vi "Query Asset Utilization.vi"(8 "Error In":errorcluster, 9 "Utilization Filter":string, 10 "Asset Filter":string, 11 "Session In":refnum<class "NI Skyline Configuration HTTP.lvclass">) -> (0 "Error Out":errorcluster, 2 "Asset Utilization":T1(array[cluster]), 3 "Session Out":refnum<class "NI Skyline Configuration HTTP.lvclass">)   [LabVIEW 2020]
uses:
  <vilib>/Skyline/Configuration/Configuration HTTP_class/NI Skyline Configuration HTTP.lvclass
  <vilib>/Skyline/Configuration/Configuration HTTP_class/NI Skyline Configuration HTTP.lvclass/NI Skyline Configuration HTTP.ctl
  <vilib>/Skyline/Configuration/Configuration HTTP_class/Read Server URL.vi
  <vilib>/httpClient/POSTBuffer.vi
  <vilib>/httpClient/LabVIEWHTTPClient.lvlib
panel:
  out "Server URL":string
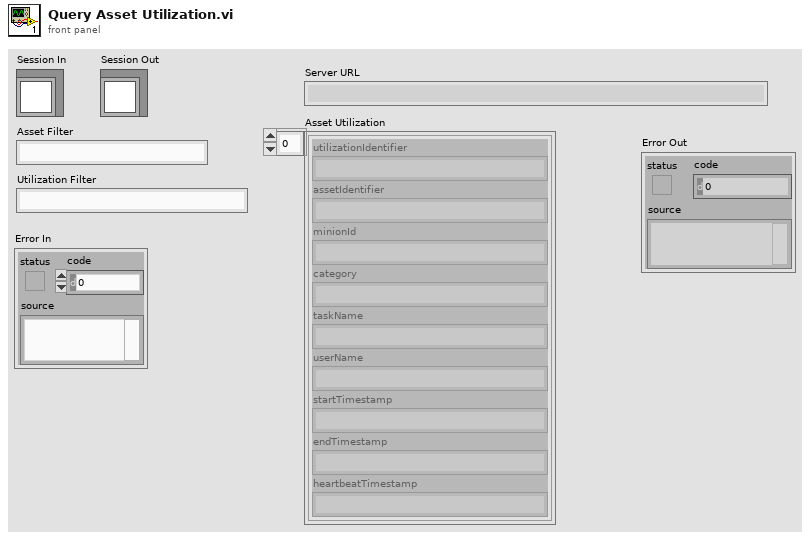
[diagram p1: front panel]
types:
  T1 = cluster{"utilizationIdentifier":string, "assetIdentifier":string, "minionId":string, "category":string, "taskName":string, "userName":string, "startTimestamp":string, "endTimestamp":string, "heartbeatTimestamp":string}[]
  T2 = cluster{"assetUtilizations":cluster{"utilizationIdentifier":string, "assetIdentifier":string, "minionId":string, "category":string, "taskName":string, "userName":string, "startTimestamp":string, "endTimestamp":string, "heartbeatTimestamp":string}[]}
  T3 = typedef "LabVIEWHTTPClient.lvlib/ClientHandle.ctl" = refnum<k1>
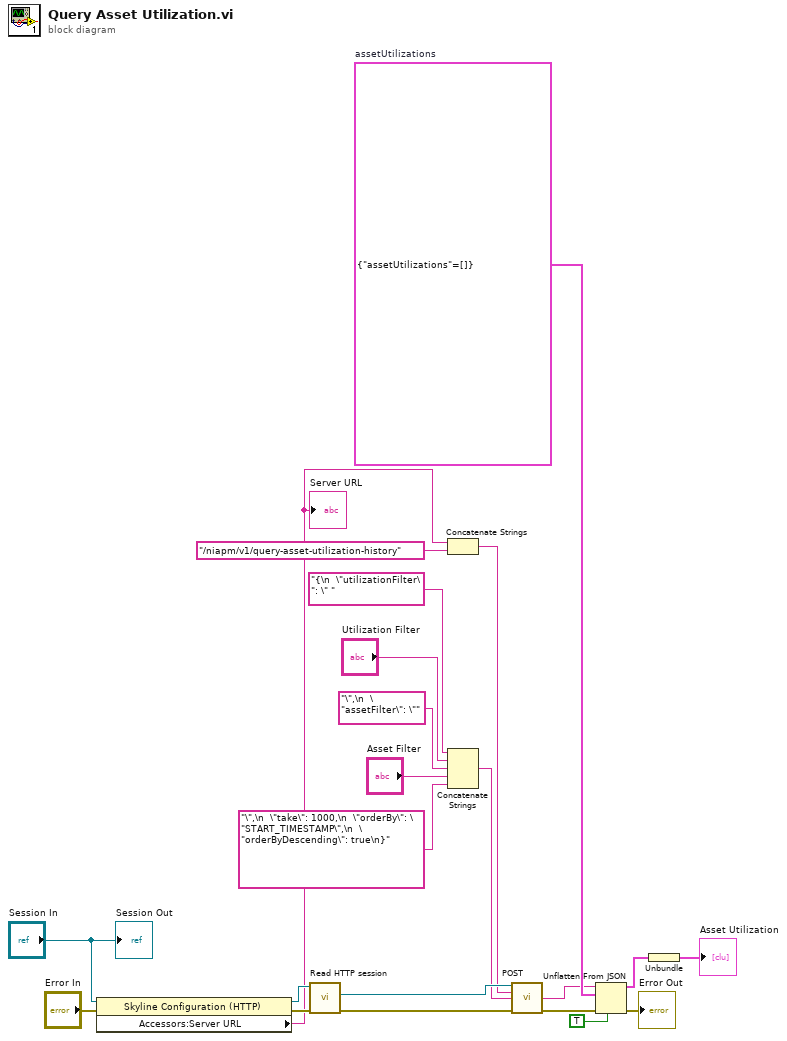
[diagram p0: block diagram]
diagram:
  w9 = T2 {"assetUtilizations"=[]}  # assetUtilizations
  n1 = property class="Skyline Configuration (HTTP)"(reference="Session In", error in="Error In") -> (reference out=w21:refnum<class "NI Skyline Configuration HTTP.lvclass">, error out=w20:errorcluster, "Accessors:Server URL"=w18:string)
  "Server URL" <- w18
  n2 = call <vilib>:"Read HTTP session.vi"("error in (no error)"=w20, "HTTP configuration in"=w21) -> ("error out"=w19:errorcluster, "http session"=w22:T3)  [unwired: 7 in, 1 out]
  n3 = Concatenate Strings(w18, "/niapm/v1/query-asset-utilization-history" ("string")) -> (w17:string)
  n4 = Concatenate Strings("{\n  \"utilizationFilter\": \" " ("buffer"), "Utilization Filter", "\",\n  \"assetFilter\": \"" ("string"), "Asset Filter", "\",\n  \"take\": 1000,\n  \"orderBy\": \"START_TIMESTAMP\",\n  \"orderByDescending\": true\n}" ("buffer")) -> (w14:string)
  n5 = call-poly <vilib>:"POST.vi"("client handle"=w22, "url"=w17, "buffer"=w14, "error in (no error)"=w19) -> ("body"=w6:string, "error out"=w2:errorcluster)  [unwired: 8 in, 2 out]
  n6 = Unflatten From JSON(JSON string=w6, type and defaults=w9, default null elements? (F)=TRUE, error in (no error)=w2) -> (value=w5:T2, error out=→"Error Out":errorcluster)  [unwired: 3 in]
  n7 = Unbundle(w5) -> ("assetUtilizations"=→"Asset Utilization":T1)
  "Session Out" <- "Session In"
